vi "Configure Power Attenuation.vi"(6 "Power Attenuation Range (0)":i32, 7 "Auto Attenuation (F: Disabled)":bool, 8 "error in (no error)":errorcluster, 9 "Port ( 1)":i32=1, 10 "Channel (1)":i32=1, 11 "VISA resource name":refnum<visa-resource-name>) -> (0 "error out":errorcluster, 3 "VISA resource name out":refnum<visa-resource-name>)   [LabVIEW 2020, in "Agilent ENA Series.lvlib"]
doc: "Configures the power settings for the instrument.\n\nNote:\nValid for E5072A only."
uses:
  <instrlib>/Agilent ENA Series/Agilent ENA Series.lvlib
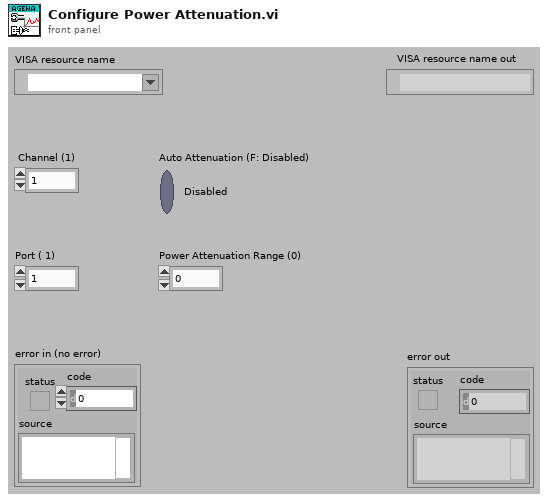
[diagram p1: front panel]
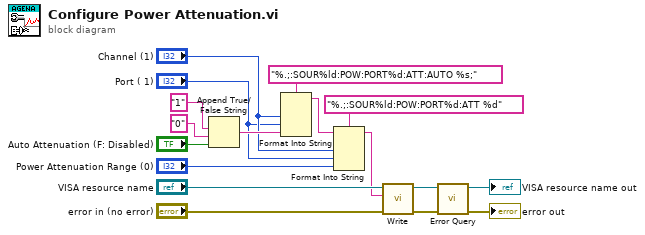
[diagram p0: block diagram]
diagram:
  n1 = Append True/False String(1:"Auto Attenuation (F: Disabled)", 2:"0" ("false string"), 3:"1" ("true string")) -> (0:w5:string)  [unwired: 1 in]
  n2 = Format Into String(format string="%.;:SOUR%ld:POW:PORT%d:ATT:AUTO %s;", "Channel (1)", "Port ( 1)", w5) -> (resulting string=w8:string)  [unwired: 2 in, 1 out]
  n3 = Format Into String(format string="%.;:SOUR%ld:POW:PORT%d:ATT %d", initial string=w8, "Channel (1)", "Port ( 1)", "Power Attenuation Range (0)") -> (resulting string=w10:string)  [unwired: 1 in, 1 out]
  n4 = call <instrlib>:"Write.vi"("error in (no error)"="error in (no error)", "String ()"=w10, "VISA resource name"="VISA resource name") -> ("error out"=w15:errorcluster, "VISA resource name out"=w14:refnum<visa-resource-name>)  [unwired: 6 in, 1 out]
  n5 = call <instrlib>:"Error Query.vi"("error in (no error)"=w15, "VISA resource name"=w14) -> ("error out"=→"error out":errorcluster, "VISA resource name out"=→"VISA resource name out":refnum<visa-resource-name>)  [unwired: 6 in, 2 out]
